vi "create_file_name.vi"(9 "File format":string=".avi", 10 "file name":string="-fish-tracking", 11 "Folder to record video":path=path "F:/") -> (3 "路径":path)   [LabVIEW 2018]
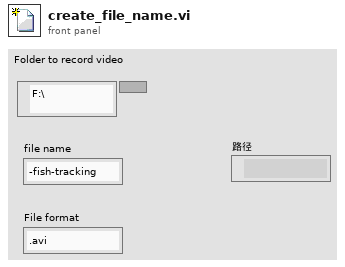
[diagram p1: front panel]
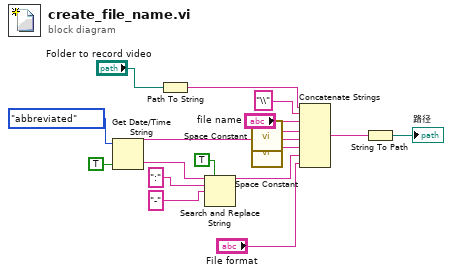
[diagram p0: block diagram]
diagram:
  n1 = Get Date/Time String(date format (0)=enum16{"short", "long", "abbreviated"}."abbreviated", want seconds? (F)=TRUE) -> (date string=w4:string, time string=w15:string)  [unwired: 1 in]
  n2 = Path To String(path="Folder to record video") -> (string=w10:string)
  n3 = Search and Replace String(replace all?=TRUE ("replace all? (F)"), input string=w15, search string=":" ("replace string (\"\")"), replace string="-" ("replace string (\"\")")) -> (result string=w2:string)  [unwired: 4 in, 3 out]
  n4 = call <vilib>:"Space Constant.vi"() -> ("String"=w5:string)
  n5 = call <vilib>:"Space Constant.vi"() -> ("String"=w3:string)
  n6 = Concatenate Strings(w10, "\\" ("string"), "file name", w5, w4, w3, w2, "File format") -> (w11:string)
  n7 = String To Path(string=w11) -> (path=→"路径":path)
